vi "GOMDBTS2048 small sample.vi"() -> ()   [LabVIEW 2009]
panel:
  out "XY Graph":cluster{i32, dbl}[](graph)
  in  "Boolean":bool
  in  "int. Time / ms":dbl
  in  "offset Mode":i32
  in  "dynamic time mode":bool
  in  "select calibration entry":string(combo)="0"
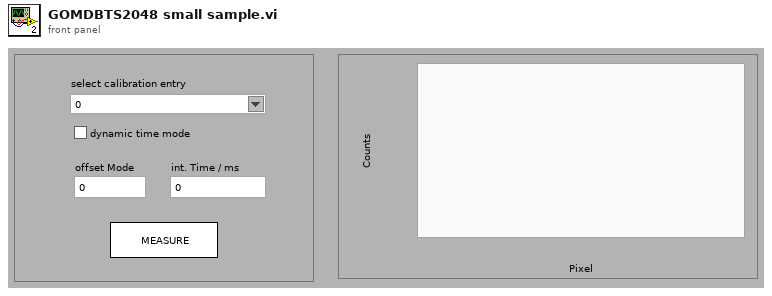
[diagram p1: front panel]
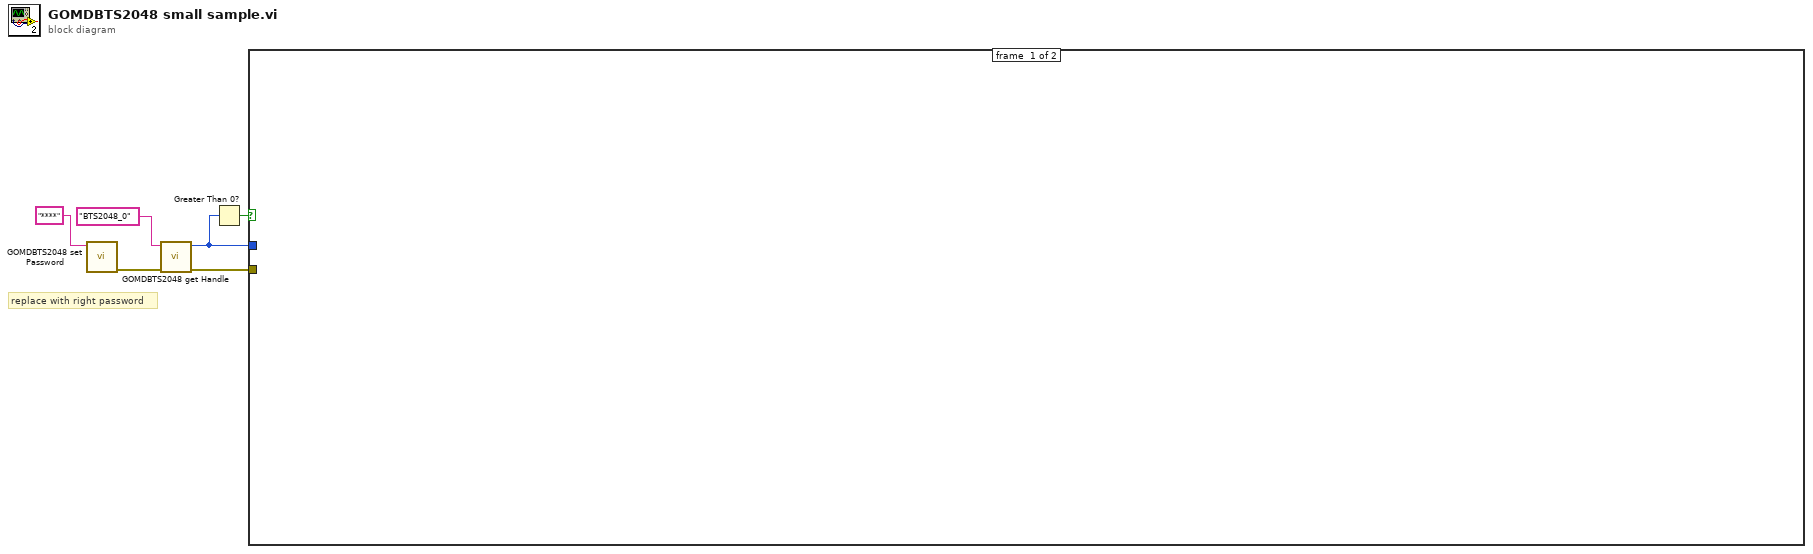
[diagram p0: block diagram]
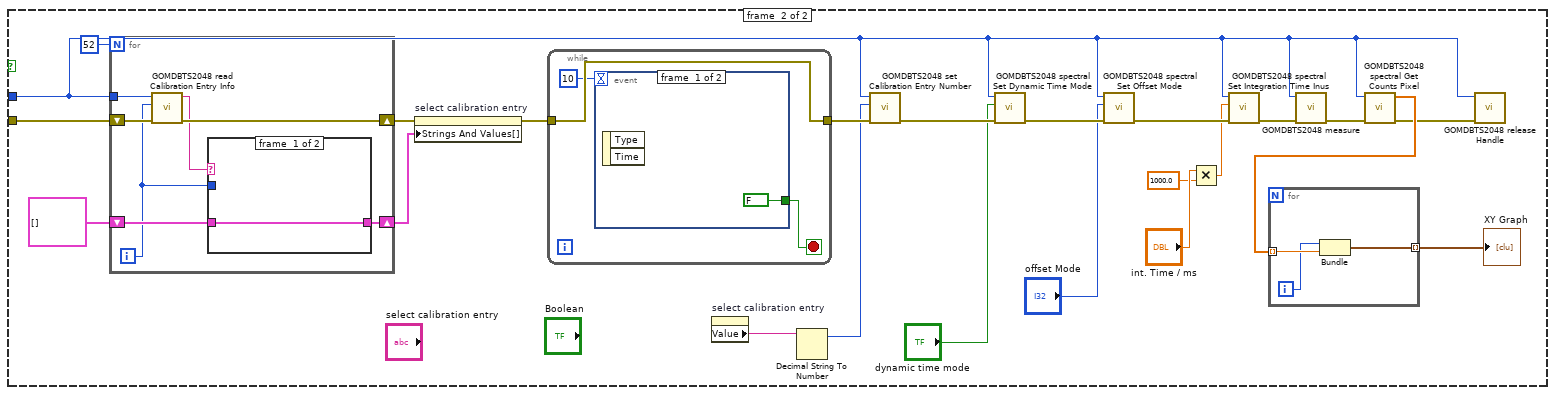
[diagram p2: hidden frame]
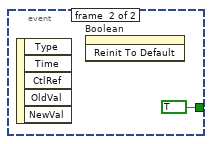
[diagram p3: hidden frame]
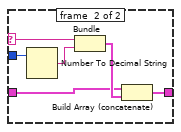
[diagram p4: hidden frame]
diagram:
  # "replace with right password"
  n1 = call <userlib>:"GOMDBTS2048 set Password.vi"("value"="****" ("deviceName")) -> ("error out"=w5:errorcluster)  [unwired: 9 in, 1 out]
  n2 = call <userlib>:"GOMDBTS2048 get Handle.vi"("error in (no error)"=w5, "device"="BTS2048_0" ("deviceName")) -> ("error out"=w4:errorcluster, "handle"=w1:i32)  [unwired: 7 in, 1 out]
  n3 = Greater Than 0?(x=w1) -> (x > 0?=w6:bool)
  n4 = case shown="True" w6 {
    tunnel: w4 -> [_ w29]
    tunnel: w1 -> [_ w8]
    frame #0 {
    }
    frame #1 {
      n5 = for {
        N: 52 -> [_]
        tunnel: w8 -> [w40]
        shift-right: [w42] -> w26
        shift-left: w29 -> [w41]
        shift-right: [w44] -> w27
        shift-left: cluster{string, string}[] [] -> [w43]
        i -> [w39]
        n6 = call <userlib>:"GOMDBTS2048 read Calibration Entry Info.vi"("error in (no error)"=w41, "calibrationEntryNumber"=w39, "handle"=w40) -> ("error out"=w42:errorcluster, "calibrationName"=w38:string)  [unwired: 6 in, 1 out]
        n7 = case shown="\"\", \"no valid entry\"" w38 {
          selector: w38 -> [_ w51]
          tunnel: w39 -> [_ w50]
          tunnel: [w45 w47] -> w44
          tunnel: w43 -> [w45 w46]
          frame #0 {
          }
          frame #1 {
            n8 = Number To Decimal String(number=w50) -> (decimal integer string=w49:string)  [unwired: 1 in]
            n9 = Bundle(w51, w49) -> (w48:cluster{string, string})  [unwired: 1 in]
            n10 = Build Array (concatenate)(w46, w48) -> (w47:cluster{string, string}[])
          }
        }
      }
      n11 = property on="select calibration entry" class="CmbBox"(error in=w26, "Strings And Values[]"=w27) -> (error out=w25:errorcluster)  [unwired: 1 in, 1 out]
      n12 = while {
        tunnel: w25 -> [w34]
        tunnel: [w34] -> w23
        stop <- w35 stop-if-true
        n13 = event shown="[1] \"Boolean\": Value Change" {
          selector: _ -> [_ _]
          dyn-events: _ -> [_ _]
          timeout: 10 -> [_ _]
          tunnel: [FALSE TRUE] -> w35
          event #0 {
            n14 = event-data() -> ()  [unwired: 1 in, 2 out]
          }
          event #1 {
            n15 = event-data() -> ()  [unwired: 1 in, 5 out]
            n16 = invoke on="Boolean" class="Bool" method="Reinit To Default"() -> ()  [unwired: 3 in, 3 out]
          }
        }
      }
      n17 = property on="select calibration entry" class="CmbBox"() -> ("Value"=w17:string)  [unwired: 2 in, 2 out]
      n18 = Decimal String To Number(string=w17) -> (offset past number=w16:i32)  [unwired: 2 in, 1 out]
      n19 = call <userlib>:"GOMDBTS2048 set Calibration Entry Number.vi"("error in (no error)"=w23, "calibrationEntryNumber"=w16, "handle"=w8) -> ("error out"=w22:errorcluster)  [unwired: 7 in, 1 out]
      n20 = call <userlib>:"GOMDBTS2048 spectral Set Dynamic Time Mode.vi"("error in (no error)"=w22, "value"="dynamic time mode", "handle"=w8) -> ("error out"=w21:errorcluster)  [unwired: 7 in, 1 out]
      n21 = call <userlib>:"GOMDBTS2048 spectral Set Offset Mode.vi"("error in (no error)"=w21, "value"="offset Mode", "handle"=w8) -> ("error out"=w20:errorcluster)  [unwired: 7 in, 1 out]
      n22 = Multiply(x="int. Time / ms", y=1000.0) -> (x*y=w13:dbl)
      n23 = call <userlib>:"GOMDBTS2048 spectral Set Integration Time Inus.vi"("error in (no error)"=w20, "timeInus"=w13, "handle"=w8) -> ("error out"=w12:errorcluster)  [unwired: 7 in, 1 out]
      n24 = call <userlib>:"GOMDBTS2048 measure.vi"("error in (no error)"=w12, "handle"=w8) -> ("error out"=w11:errorcluster)  [unwired: 8 in, 1 out]
      n25 = call <userlib>:"GOMDBTS2048 spectral Get Counts Pixel.vi"("error in (no error)"=w11, "handle"=w8) -> ("error out"=w7:errorcluster, "counts"=w9:dbl[])  [unwired: 7 in, 1 out]
      n26 = for {
        tunnel: w9 -> [w32] mode=indexing
        tunnel: [w30] -> w10 mode=indexing
        i -> [w31]
        n27 = Bundle(w31, w32) -> (w30:cluster{i32, dbl})  [unwired: 1 in]
      }
      "XY Graph" <- w10
      n28 = call <userlib>:"GOMDBTS2048 release Handle.vi"("error in (no error)"=w7, "handle"=w8) -> ()  [unwired: 8 in, 2 out]
    }
  }
